vi "BRig_dataCurrent_idxDataBlock.vi"() -> (2 "output_idxDataBlock":i32)   [LabVIEW 2014]
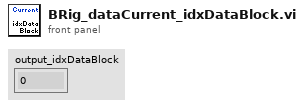
[diagram p1: front panel]
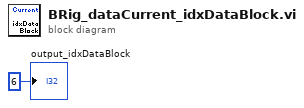
[diagram p0: block diagram]
diagram:
  "output_idxDataBlock" <- 6 ("output_iBlock")
